vi "总磷氨氮测量数据储存.vi"   [LabVIEW 2016, in "斯坦道仪器.lvlib"]
types:
  T1 = enum16{"维护数据", "水样测试", "标样核查", "零点核查", "跨度核查", "空白测试", "平行样测试", "加标回收", "空白校准", "标样校准", "初始化（清洗）"}
  T2 = cluster{"时间标识":timestamp, "监测值":sgl, "单位":u16, "数据标识":string, "因子编码":u32, "标样参考值":sgl, "F0":sgl, "F1":sgl, "F2":sgl, "F3":sgl, "温度":sgl, "湿度":sgl, "量程标识":string}
  T3 = cluster{"系统时间":timestamp, "工作状态":enum16{"空闲", "水样测试", "标样核查", "零点核查", "跨度核查", "空白测试", "平行样测试", "加标回收", "空白校准", "标样校准", "初始化（清洗）"}, "测量模式":enum16{"待机", "连续模式", "周期模式", "定点模式", "受控模式", "手动模式"}, "告警代码":enum16{"无告警", "缺试剂告警", "缺水样告警", "缺蒸馏水告警", "缺标液告警", "仪表漏液告警", "标定异常告警", "超量程告警", "加热异常", "低试剂预警", "超上限告警", "超下限告警", "仪表内部其他异常", "滴定异常告警", "电极异常告警", "量程切换告警", "参数设置告警", "PH电极电位异常", "电导率电极异常", "浊度光度异常", "溶解氧电极异常", "溶解氧光强异常", "温度异常告警", "PH异常告警", "溶解氧异常告警", "电导率异常告警", "浊度异常告警", "叶绿素异常告警", "藻密度异常告警", "蓝绿藻异常告警", "ORP异常告警", "氨氮异常告警", "清洁刷异常告警", "SD卡异常告警", "蓝牙异常告警", "Wifi异常告警", "流程异常告警"}, "故障代码":enum16{"无故障", "电机故障", "温度故障", "通讯故障", "滴定故障"}, "日志代码":u16, "软件版本":u16, "F0":sgl, "F1":sgl, "F2":sgl, "F3":sgl, "T":sgl, "H":sgl, "id":u16, "flowid":u16, "量程":u16}
  T4 = enum16{"空闲", "水样测试", "标样核查", "零点核查", "跨度核查", "空白测试", "平行样测试", "加标回收", "空白校准", "标样校准", "初始化（清洗）"}
  T5 = cluster{"因子编码":u32, "单位":u16, "标样参考值":sgl, "水样数据时间":timestamp, "水样实测值":sgl, "水样数据标识":string, "标样数据时间":timestamp, "标样实测值":sgl, "标样数据标识":string, "空白数据时间":timestamp, "空白实测值":sgl, "空白数据标识":string, "零点核查数据时间":timestamp, "零点核查实测值":sgl, "零点核查数据标识":string, "跨度核查数据时间":timestamp, "跨度核查实测值":sgl, "跨度核查数据标识":string, "加标回收数据时间":timestamp, "加标回收实测值":sgl, "加标回收数据标识":string, "平行样数据时间":timestamp, "平行样实测值":sgl, "平行样数据标识":string}
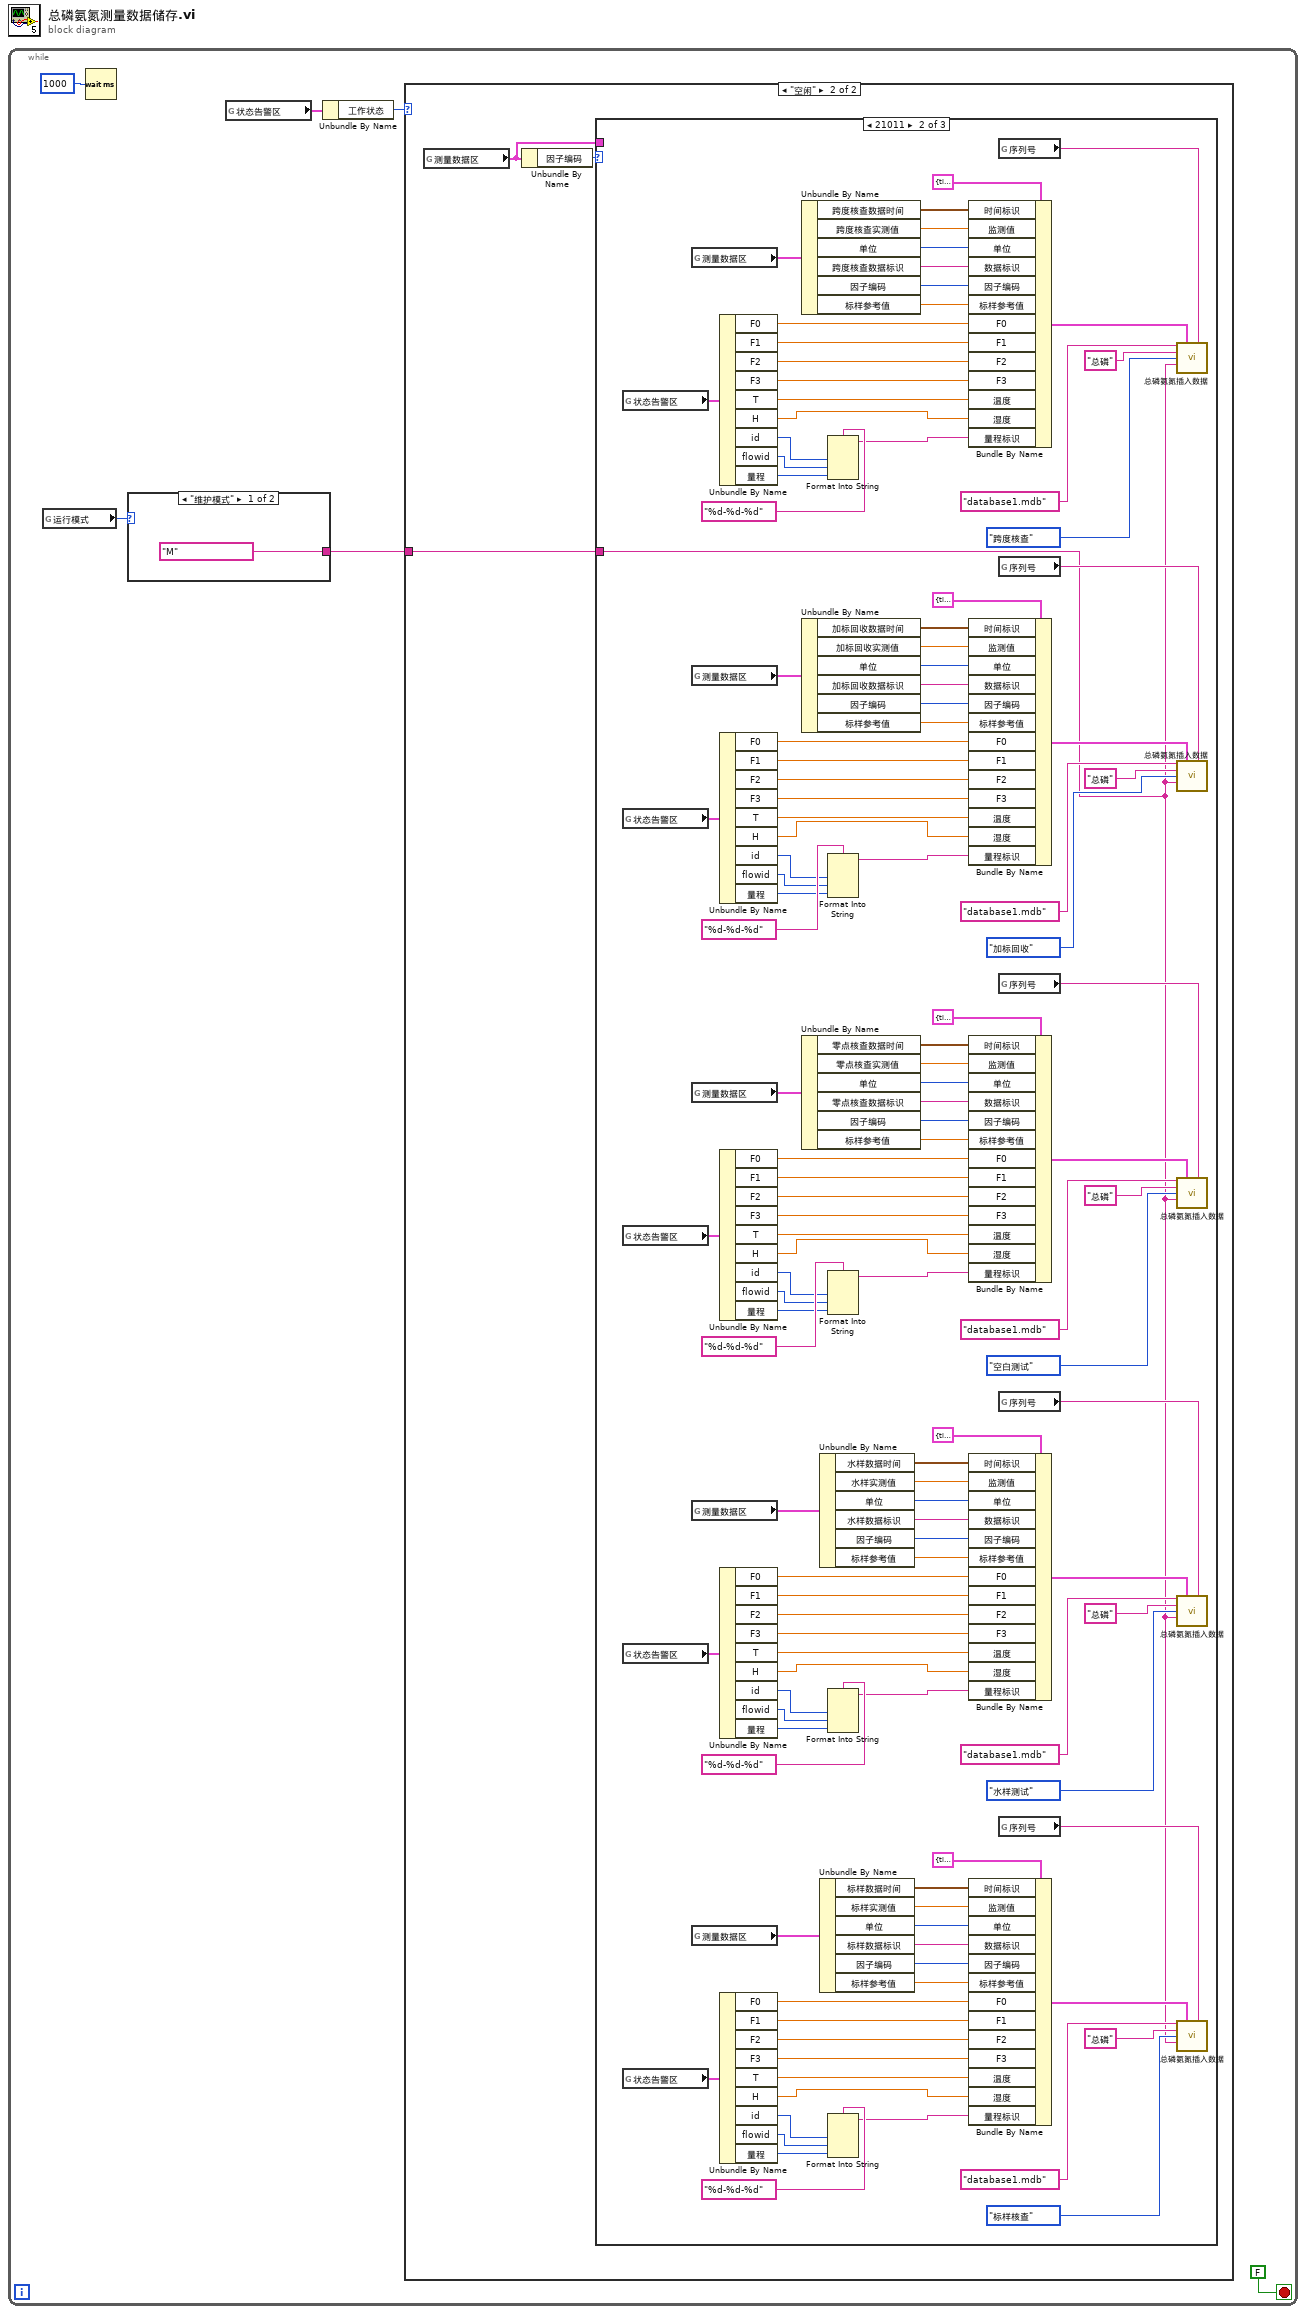
[diagram p0: block diagram]
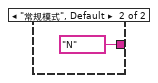
[diagram p2: hidden frame]
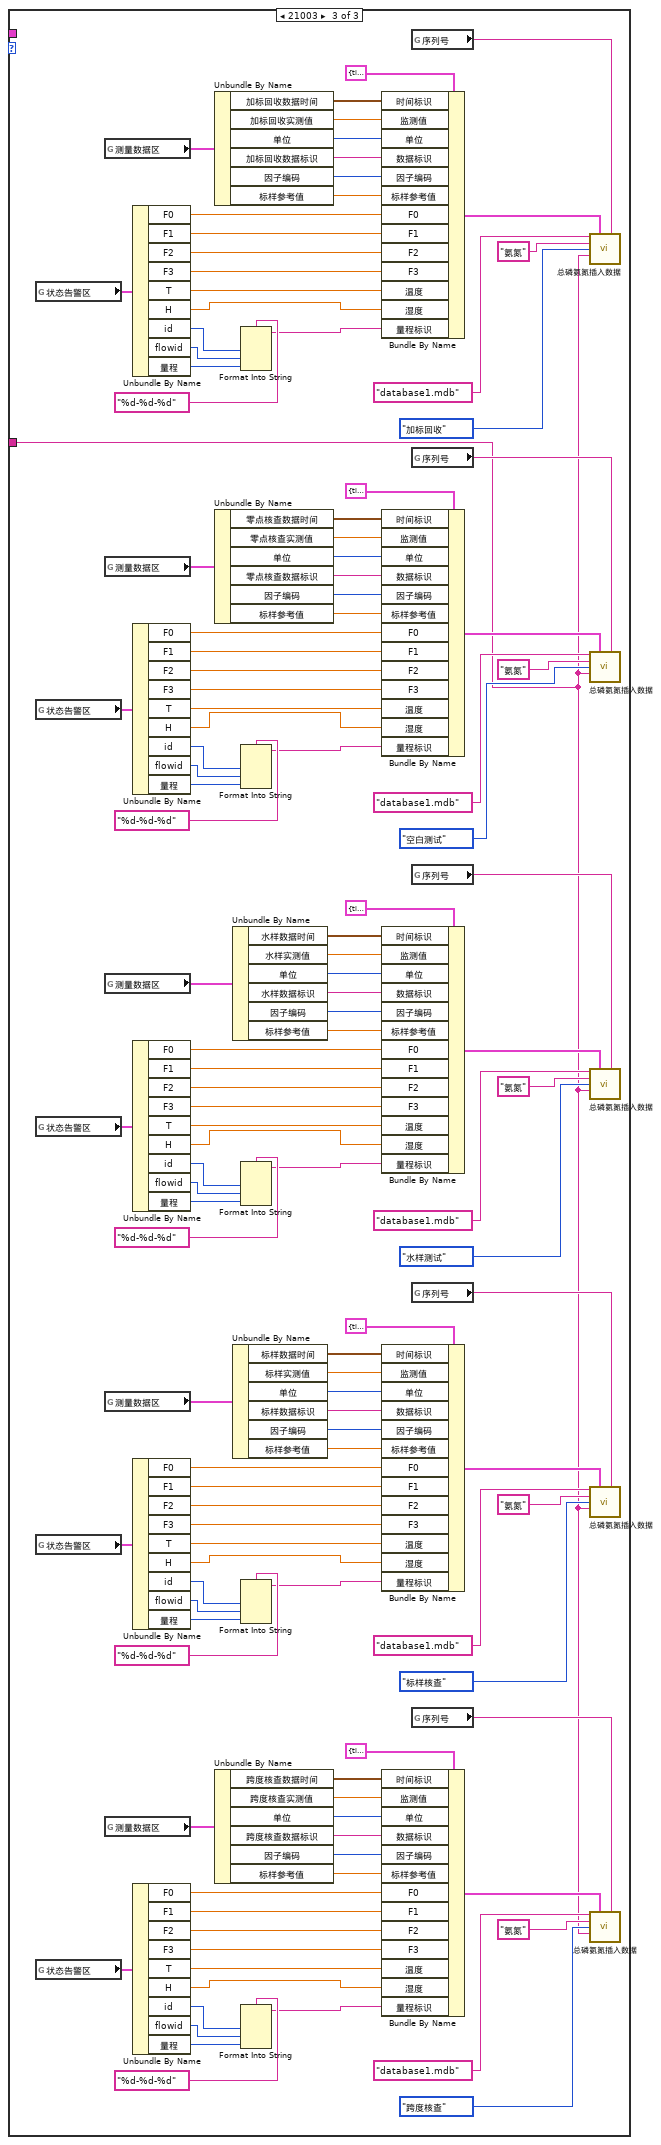
[diagram p5: hidden frame]
diagram:
  n1 = while {
    stop <- FALSE stop-if-true
    n2 = global read "系统变量.vi" "运行模式"() -> (w2:enum16{"维护模式", "常规模式", "应急模式", "质控模式"})
    n3 = Wait (ms)(milliseconds to wait=u32 1000 ("等待时间（毫秒）")) -> ()  [unwired: 1 out]
    n4 = case shown="\"维护模式\"" w2 {
      tunnel: ["M" ("数据标记表") "N" ("数据标记表")] -> w1
      frame "维护模式" {
      }
      frame "常规模式", Default {
      }
    }
    n5 = global read "VAR总磷氨氮全局变量.vi" "状态告警区"() -> (w4:T3)
    n6 = Unbundle By Name(w4) -> ("工作状态"=w3:T4)
    n7 = case shown="\"空闲\"" w3 {
      tunnel: w1 -> [_ w9]
      frame Default {
      }
      frame "空闲" {
        n8 = global read "VAR总磷氨氮全局变量.vi" "测量数据区"() -> (w11:T5)
        n9 = Unbundle By Name(w11) -> ("因子编码"=w10:u32)
        n10 = case shown="21011" w10 {
          tunnel: w11 -> [_ _ _]
          tunnel: w9 -> [_ w12 w138]
          frame Default {
          }
          frame 21011 {
            n11 = global read "VAR总磷氨氮全局变量.vi" "状态告警区"() -> (w76:T3)
            n12 = global read "VAR总磷氨氮全局变量.vi" "状态告警区"() -> (w58:T3)
            n13 = global read "VAR总磷氨氮全局变量.vi" "状态告警区"() -> (w91:T3)
            n14 = global read "VAR总磷氨氮全局变量.vi" "状态告警区"() -> (w130:T3)
            n15 = global read "VAR总磷氨氮全局变量.vi" "状态告警区"() -> (w109:T3)
            n16 = global read "VAR总磷氨氮全局变量.vi" "测量数据区"() -> (w83:T5)
            n17 = global read "VAR总磷氨氮全局变量.vi" "测量数据区"() -> (w65:T5)
            n18 = global read "VAR总磷氨氮全局变量.vi" "测量数据区"() -> (w84:T5)
            n19 = global read "VAR总磷氨氮全局变量.vi" "测量数据区"() -> (w137:T5)
            n20 = global read "VAR总磷氨氮全局变量.vi" "测量数据区"() -> (w102:T5)
            n21 = Unbundle By Name(w76) -> ("F0"=w75:sgl, "F1"=w74:sgl, "F2"=w73:sgl, "F3"=w72:sgl, "T"=w71:sgl, "H"=w70:sgl, "id"=w39:u16, "flowid"=w38:u16, "量程"=w37:u16)
            n22 = Unbundle By Name(w58) -> ("F0"=w57:sgl, "F1"=w56:sgl, "F2"=w55:sgl, "F3"=w54:sgl, "T"=w53:sgl, "H"=w52:sgl, "id"=w45:u16, "flowid"=w44:u16, "量程"=w43:u16)
            n23 = Unbundle By Name(w91) -> ("F0"=w92:sgl, "F1"=w93:sgl, "F2"=w94:sgl, "F3"=w95:sgl, "T"=w96:sgl, "H"=w97:sgl, "id"=w32:u16, "flowid"=w33:u16, "量程"=w34:u16)
            n24 = Unbundle By Name(w130) -> ("F0"=w129:sgl, "F1"=w128:sgl, "F2"=w127:sgl, "F3"=w126:sgl, "T"=w125:sgl, "H"=w124:sgl, "id"=w19:u16, "flowid"=w20:u16, "量程"=w21:u16)
            n25 = Unbundle By Name(w109) -> ("F0"=w110:sgl, "F1"=w111:sgl, "F2"=w112:sgl, "F3"=w113:sgl, "T"=w114:sgl, "H"=w115:sgl, "id"=w27:u16, "flowid"=w26:u16, "量程"=w25:u16)
            n26 = Unbundle By Name(w83) -> ("跨度核查数据时间"=w82:timestamp, "跨度核查实测值"=w81:sgl, "单位"=w80:u16, "跨度核查数据标识"=w79:string, "因子编码"=w78:u32, "标样参考值"=w77:sgl)
            n27 = Unbundle By Name(w65) -> ("加标回收数据时间"=w64:timestamp, "加标回收实测值"=w63:sgl, "单位"=w62:u16, "加标回收数据标识"=w61:string, "因子编码"=w60:u32, "标样参考值"=w59:sgl)
            n28 = Unbundle By Name(w84) -> ("零点核查数据时间"=w85:timestamp, "零点核查实测值"=w86:sgl, "单位"=w87:u16, "零点核查数据标识"=w88:string, "因子编码"=w89:u32, "标样参考值"=w90:sgl)
            n29 = Unbundle By Name(w137) -> ("水样数据时间"=w136:timestamp, "水样实测值"=w135:sgl, "单位"=w134:u16, "水样数据标识"=w133:string, "因子编码"=w132:u32, "标样参考值"=w131:sgl)
            n30 = Unbundle By Name(w102) -> ("标样数据时间"=w103:timestamp, "标样实测值"=w104:sgl, "单位"=w105:u16, "标样数据标识"=w106:string, "因子编码"=w107:u32, "标样参考值"=w108:sgl)
            n31 = Format Into String(format string="%d-%d-%d" ("格式字符串"), w39, w38, w37) -> (resulting string=w36:string)  [unwired: 2 in, 1 out]
            n32 = Format Into String(format string="%d-%d-%d" ("格式字符串"), w45, w44, w43) -> (resulting string=w42:string)  [unwired: 2 in, 1 out]
            n33 = Format Into String(format string="%d-%d-%d" ("格式字符串"), w32, w33, w34) -> (resulting string=w30:string)  [unwired: 2 in, 1 out]
            n34 = Format Into String(format string="%d-%d-%d" ("格式字符串"), w19, w20, w21) -> (resulting string=w18:string)  [unwired: 2 in, 1 out]
            n35 = Format Into String(format string="%d-%d-%d" ("格式字符串"), w27, w26, w25) -> (resulting string=w24:string)  [unwired: 2 in, 1 out]
            n36 = Bundle By Name(cluster=T2 {"时间标识"=timestamp(0 s since 1904-01-01), "监测值"=0.0, "单位"=0, "数据标识"="", "因子编码"=0, "标样参考值"=0.0, "F0"=0.0, "F1"=0.0, "F2"=0.0, "F3"=0.0, "温度"=0.0, "湿度"=0.0, "量程标识"=""} ("data"), "时间标识"=w82, "监测值"=w81, "单位"=w80, "数据标识"=w79, "因子编码"=w78, "标样参考值"=w77, "F0"=w75, "F1"=w74, "F2"=w73, "F3"=w72, "温度"=w71, "湿度"=w70, "量程标识"=w36) -> (w69:T2)
            n37 = Bundle By Name(cluster=T2 {"时间标识"=timestamp(0 s since 1904-01-01), "监测值"=0.0, "单位"=0, "数据标识"="", "因子编码"=0, "标样参考值"=0.0, "F0"=0.0, "F1"=0.0, "F2"=0.0, "F3"=0.0, "温度"=0.0, "湿度"=0.0, "量程标识"=""} ("data"), "时间标识"=w64, "监测值"=w63, "单位"=w62, "数据标识"=w61, "因子编码"=w60, "标样参考值"=w59, "F0"=w57, "F1"=w56, "F2"=w55, "F3"=w54, "温度"=w53, "湿度"=w52, "量程标识"=w42) -> (w51:T2)
            n38 = Bundle By Name(cluster=T2 {"时间标识"=timestamp(0 s since 1904-01-01), "监测值"=0.0, "单位"=0, "数据标识"="", "因子编码"=0, "标样参考值"=0.0, "F0"=0.0, "F1"=0.0, "F2"=0.0, "F3"=0.0, "温度"=0.0, "湿度"=0.0, "量程标识"=""} ("data"), "时间标识"=w85, "监测值"=w86, "单位"=w87, "数据标识"=w88, "因子编码"=w89, "标样参考值"=w90, "F0"=w92, "F1"=w93, "F2"=w94, "F3"=w95, "温度"=w96, "湿度"=w97, "量程标识"=w30) -> (w98:T2)
            n39 = Bundle By Name(cluster=T2 {"时间标识"=timestamp(0 s since 1904-01-01), "监测值"=0.0, "单位"=0, "数据标识"="", "因子编码"=0, "标样参考值"=0.0, "F0"=0.0, "F1"=0.0, "F2"=0.0, "F3"=0.0, "温度"=0.0, "湿度"=0.0, "量程标识"=""} ("data"), "时间标识"=w136, "监测值"=w135, "单位"=w134, "数据标识"=w133, "因子编码"=w132, "标样参考值"=w131, "F0"=w129, "F1"=w128, "F2"=w127, "F3"=w126, "温度"=w125, "湿度"=w124, "量程标识"=w18) -> (w123:T2)
            n40 = Bundle By Name(cluster=T2 {"时间标识"=timestamp(0 s since 1904-01-01), "监测值"=0.0, "单位"=0, "数据标识"="", "因子编码"=0, "标样参考值"=0.0, "F0"=0.0, "F1"=0.0, "F2"=0.0, "F3"=0.0, "温度"=0.0, "湿度"=0.0, "量程标识"=""} ("data"), "时间标识"=w103, "监测值"=w104, "单位"=w105, "数据标识"=w106, "因子编码"=w107, "标样参考值"=w108, "F0"=w110, "F1"=w111, "F2"=w112, "F3"=w113, "温度"=w114, "湿度"=w115, "量程标识"=w24) -> (w116:T2)
            n41 = global read "VAR总磷氨氮全局变量.vi" "序列号"() -> (w14:string)
            n42 = global read "VAR总磷氨氮全局变量.vi" "序列号"() -> (w13:string)
            n43 = global read "VAR总磷氨氮全局变量.vi" "序列号"() -> (w15:string)
            n44 = global read "VAR总磷氨氮全局变量.vi" "序列号"() -> (w17:string)
            n45 = global read "VAR总磷氨氮全局变量.vi" "序列号"() -> (w16:string)
            n46 = call "总磷氨氮插入数据.vi"("database"="database1.mdb", "data"=w69, "SN"=w14, "table"="总磷", "测量模式"=T1."跨度核查", "数据标记表"=w12) -> ()  [unwired: 9 in, 1 out]
            n47 = call "总磷氨氮插入数据.vi"("database"="database1.mdb", "data"=w51, "SN"=w13, "table"="总磷", "测量模式"=T1."加标回收", "数据标记表"=w12) -> ()  [unwired: 9 in, 1 out]
            n48 = call "总磷氨氮插入数据.vi"("database"="database1.mdb", "data"=w98, "SN"=w15, "table"="总磷", "测量模式"=T1."空白测试", "数据标记表"=w12) -> ()  [unwired: 9 in, 1 out]
            n49 = call "总磷氨氮插入数据.vi"("database"="database1.mdb", "data"=w123, "SN"=w17, "table"="总磷", "测量模式"=T1."水样测试", "数据标记表"=w12) -> ()  [unwired: 9 in, 1 out]
            n50 = call "总磷氨氮插入数据.vi"("database"="database1.mdb", "data"=w116, "SN"=w16, "table"="总磷", "测量模式"=T1."标样核查", "数据标记表"=w12) -> ()  [unwired: 9 in, 1 out]
          }
          frame 21003 {
            n51 = global read "VAR总磷氨氮全局变量.vi" "状态告警区"() -> (w184:T3)
            n52 = global read "VAR总磷氨氮全局变量.vi" "状态告警区"() -> (w217:T3)
            n53 = global read "VAR总磷氨氮全局变量.vi" "状态告警区"() -> (w256:T3)
            n54 = global read "VAR总磷氨氮全局变量.vi" "状态告警区"() -> (w235:T3)
            n55 = global read "VAR总磷氨氮全局变量.vi" "状态告警区"() -> (w202:T3)
            n56 = global read "VAR总磷氨氮全局变量.vi" "测量数据区"() -> (w191:T5)
            n57 = global read "VAR总磷氨氮全局变量.vi" "测量数据区"() -> (w210:T5)
            n58 = global read "VAR总磷氨氮全局变量.vi" "测量数据区"() -> (w263:T5)
            n59 = global read "VAR总磷氨氮全局变量.vi" "测量数据区"() -> (w228:T5)
            n60 = global read "VAR总磷氨氮全局变量.vi" "测量数据区"() -> (w209:T5)
            n61 = Unbundle By Name(w184) -> ("F0"=w183:sgl, "F1"=w182:sgl, "F2"=w181:sgl, "F3"=w180:sgl, "T"=w179:sgl, "H"=w178:sgl, "id"=w159:u16, "flowid"=w158:u16, "量程"=w157:u16)
            n62 = Unbundle By Name(w217) -> ("F0"=w218:sgl, "F1"=w219:sgl, "F2"=w220:sgl, "F3"=w221:sgl, "T"=w222:sgl, "H"=w223:sgl, "id"=w147:u16, "flowid"=w146:u16, "量程"=w145:u16)
            n63 = Unbundle By Name(w256) -> ("F0"=w255:sgl, "F1"=w254:sgl, "F2"=w253:sgl, "F3"=w252:sgl, "T"=w251:sgl, "H"=w250:sgl, "id"=w172:u16, "flowid"=w171:u16, "量程"=w170:u16)
            n64 = Unbundle By Name(w235) -> ("F0"=w236:sgl, "F1"=w237:sgl, "F2"=w238:sgl, "F3"=w239:sgl, "T"=w240:sgl, "H"=w241:sgl, "id"=w165:u16, "flowid"=w164:u16, "量程"=w163:u16)
            n65 = Unbundle By Name(w202) -> ("F0"=w201:sgl, "F1"=w200:sgl, "F2"=w199:sgl, "F3"=w198:sgl, "T"=w197:sgl, "H"=w196:sgl, "id"=w153:u16, "flowid"=w152:u16, "量程"=w151:u16)
            n66 = Unbundle By Name(w191) -> ("加标回收数据时间"=w190:timestamp, "加标回收实测值"=w189:sgl, "单位"=w188:u16, "加标回收数据标识"=w187:string, "因子编码"=w186:u32, "标样参考值"=w185:sgl)
            n67 = Unbundle By Name(w210) -> ("零点核查数据时间"=w211:timestamp, "零点核查实测值"=w212:sgl, "单位"=w213:u16, "零点核查数据标识"=w214:string, "因子编码"=w215:u32, "标样参考值"=w216:sgl)
            n68 = Unbundle By Name(w209) -> ("跨度核查数据时间"=w208:timestamp, "跨度核查实测值"=w207:sgl, "单位"=w206:u16, "跨度核查数据标识"=w205:string, "因子编码"=w204:u32, "标样参考值"=w203:sgl)
            n69 = Unbundle By Name(w263) -> ("水样数据时间"=w262:timestamp, "水样实测值"=w261:sgl, "单位"=w260:u16, "水样数据标识"=w259:string, "因子编码"=w258:u32, "标样参考值"=w257:sgl)
            n70 = Unbundle By Name(w228) -> ("标样数据时间"=w229:timestamp, "标样实测值"=w230:sgl, "单位"=w231:u16, "标样数据标识"=w232:string, "因子编码"=w233:u32, "标样参考值"=w234:sgl)
            n71 = Format Into String(format string="%d-%d-%d" ("格式字符串"), w159, w158, w157) -> (resulting string=w156:string)  [unwired: 2 in, 1 out]
            n72 = Format Into String(format string="%d-%d-%d" ("格式字符串"), w147, w146, w145) -> (resulting string=w144:string)  [unwired: 2 in, 1 out]
            n73 = Format Into String(format string="%d-%d-%d" ("格式字符串"), w172, w171, w170) -> (resulting string=w168:string)  [unwired: 2 in, 1 out]
            n74 = Format Into String(format string="%d-%d-%d" ("格式字符串"), w165, w164, w163) -> (resulting string=w162:string)  [unwired: 2 in, 1 out]
            n75 = Format Into String(format string="%d-%d-%d" ("格式字符串"), w153, w152, w151) -> (resulting string=w150:string)  [unwired: 2 in, 1 out]
            n76 = Bundle By Name(cluster=T2 {"时间标识"=timestamp(0 s since 1904-01-01), "监测值"=0.0, "单位"=0, "数据标识"="", "因子编码"=0, "标样参考值"=0.0, "F0"=0.0, "F1"=0.0, "F2"=0.0, "F3"=0.0, "温度"=0.0, "湿度"=0.0, "量程标识"=""} ("data"), "时间标识"=w190, "监测值"=w189, "单位"=w188, "数据标识"=w187, "因子编码"=w186, "标样参考值"=w185, "F0"=w183, "F1"=w182, "F2"=w181, "F3"=w180, "温度"=w179, "湿度"=w178, "量程标识"=w156) -> (w177:T2)
            n77 = Bundle By Name(cluster=T2 {"时间标识"=timestamp(0 s since 1904-01-01), "监测值"=0.0, "单位"=0, "数据标识"="", "因子编码"=0, "标样参考值"=0.0, "F0"=0.0, "F1"=0.0, "F2"=0.0, "F3"=0.0, "温度"=0.0, "湿度"=0.0, "量程标识"=""} ("data"), "时间标识"=w211, "监测值"=w212, "单位"=w213, "数据标识"=w214, "因子编码"=w215, "标样参考值"=w216, "F0"=w218, "F1"=w219, "F2"=w220, "F3"=w221, "温度"=w222, "湿度"=w223, "量程标识"=w144) -> (w224:T2)
            n78 = Bundle By Name(cluster=T2 {"时间标识"=timestamp(0 s since 1904-01-01), "监测值"=0.0, "单位"=0, "数据标识"="", "因子编码"=0, "标样参考值"=0.0, "F0"=0.0, "F1"=0.0, "F2"=0.0, "F3"=0.0, "温度"=0.0, "湿度"=0.0, "量程标识"=""} ("data"), "时间标识"=w262, "监测值"=w261, "单位"=w260, "数据标识"=w259, "因子编码"=w258, "标样参考值"=w257, "F0"=w255, "F1"=w254, "F2"=w253, "F3"=w252, "温度"=w251, "湿度"=w250, "量程标识"=w168) -> (w249:T2)
            n79 = Bundle By Name(cluster=T2 {"时间标识"=timestamp(0 s since 1904-01-01), "监测值"=0.0, "单位"=0, "数据标识"="", "因子编码"=0, "标样参考值"=0.0, "F0"=0.0, "F1"=0.0, "F2"=0.0, "F3"=0.0, "温度"=0.0, "湿度"=0.0, "量程标识"=""} ("data"), "时间标识"=w229, "监测值"=w230, "单位"=w231, "数据标识"=w232, "因子编码"=w233, "标样参考值"=w234, "F0"=w236, "F1"=w237, "F2"=w238, "F3"=w239, "温度"=w240, "湿度"=w241, "量程标识"=w162) -> (w242:T2)
            n80 = Bundle By Name(cluster=T2 {"时间标识"=timestamp(0 s since 1904-01-01), "监测值"=0.0, "单位"=0, "数据标识"="", "因子编码"=0, "标样参考值"=0.0, "F0"=0.0, "F1"=0.0, "F2"=0.0, "F3"=0.0, "温度"=0.0, "湿度"=0.0, "量程标识"=""} ("data"), "时间标识"=w208, "监测值"=w207, "单位"=w206, "数据标识"=w205, "因子编码"=w204, "标样参考值"=w203, "F0"=w201, "F1"=w200, "F2"=w199, "F3"=w198, "温度"=w197, "湿度"=w196, "量程标识"=w150) -> (w195:T2)
            n81 = global read "VAR总磷氨氮全局变量.vi" "序列号"() -> (w139:string)
            n82 = global read "VAR总磷氨氮全局变量.vi" "序列号"() -> (w141:string)
            n83 = global read "VAR总磷氨氮全局变量.vi" "序列号"() -> (w143:string)
            n84 = global read "VAR总磷氨氮全局变量.vi" "序列号"() -> (w142:string)
            n85 = global read "VAR总磷氨氮全局变量.vi" "序列号"() -> (w140:string)
            n86 = call "总磷氨氮插入数据.vi"("database"="database1.mdb", "data"=w177, "SN"=w139, "table"="氨氮", "测量模式"=T1."加标回收", "数据标记表"=w138) -> ()  [unwired: 9 in, 1 out]
            n87 = call "总磷氨氮插入数据.vi"("database"="database1.mdb", "data"=w224, "SN"=w141, "table"="氨氮", "测量模式"=T1."空白测试", "数据标记表"=w138) -> ()  [unwired: 9 in, 1 out]
            n88 = call "总磷氨氮插入数据.vi"("database"="database1.mdb", "data"=w249, "SN"=w143, "table"="氨氮", "测量模式"=T1."水样测试", "数据标记表"=w138) -> ()  [unwired: 9 in, 1 out]
            n89 = call "总磷氨氮插入数据.vi"("database"="database1.mdb", "data"=w242, "SN"=w142, "table"="氨氮", "测量模式"=T1."标样核查", "数据标记表"=w138) -> ()  [unwired: 9 in, 1 out]
            n90 = call "总磷氨氮插入数据.vi"("database"="database1.mdb", "data"=w195, "SN"=w140, "table"="氨氮", "测量模式"=T1."跨度核查", "数据标记表"=w138) -> ()  [unwired: 9 in, 1 out]
          }
        }
      }
    }
  }
